vi "Create System Image (Folder).vi"(4 "File and Directory Blacklist":string[](array[string]), 5 "Encryption Passphrase":string, 6 "Overwrite (F)":bool, 7 "Restart Automatically (T)":bool=TRUE, 8 "error in (no error)":errorcluster, 9 "Image Metadata in":T1={"title"="", "description"="", "ID"="", "version"="", "component type"=5} {"component type" items=["standard", "hidden", "system", "unknown", "startup", "image"]}, 10 "Destination Folder":path, 11 "Session in":refnum<k21>) -> (0 "error out":errorcluster, 1 "Image Metadata out":T1={"title"="", "description"="", "ID"="", "version"="", "component type"=5} {"component type" items=["standard", "hidden", "system", "unknown", "startup", "image"]}, 3 "Session out":refnum<k21>)   [LabVIEW 2014, in "nisyscfg.lvlib"]
doc: "Creates a system image folder—a copy of the contents and software on a primary hard drive of a system. You may want to create a system image to restore a system to its original state or to deploy the image to other systems."
uses:
  nisyscfg.lvlib
  Software 1.2.ctl
  Component Type.ctl
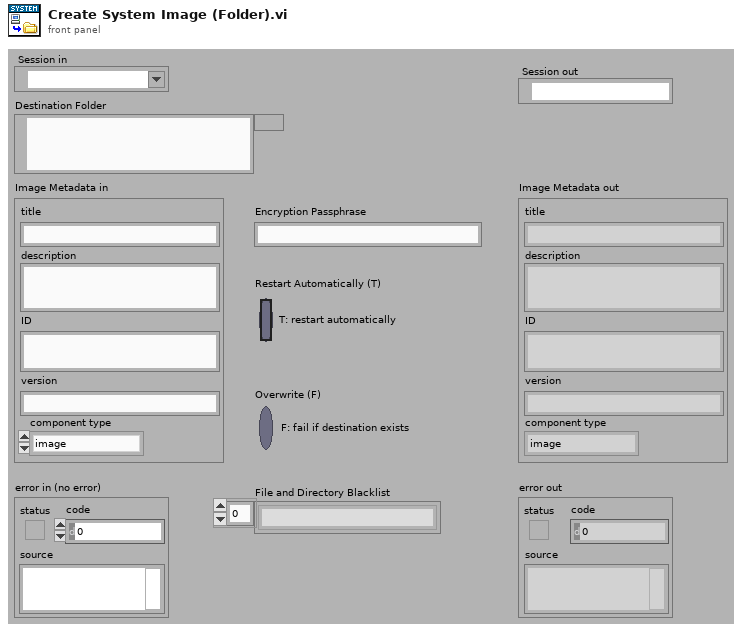
[diagram p1: front panel]
types:
  T1 = typedef "nisyscfg.lvlib/Software 1.2.ctl" = cluster{"title":string, "description":string, "ID":string, "version":string, "component type":T2}
  T2 = typedef "nisyscfg.lvlib/Component Type.ctl" = u32
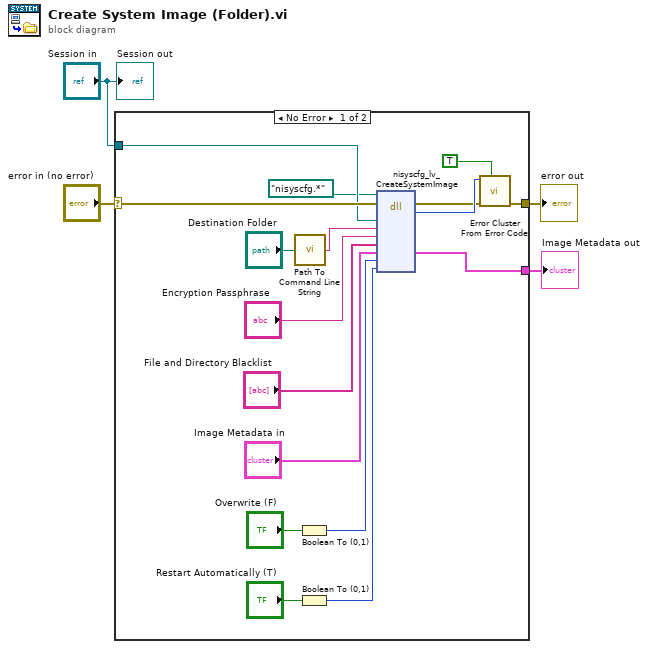
[diagram p0: block diagram]
diagram:
  n1 = case shown="No Error" "error in (no error)" {
    selector: "error in (no error)" -> [w18 w22]
    tunnel: [w21 w22] -> w4
    tunnel: "Session in" -> [w17 _]
    tunnel: [w5 _] -> w1
    frame No Error {
      n2 = call "Path To Command Line String.vi"("path"="Destination Folder") -> ("string"=w7:string)
      n3 = Boolean To (0,1)(Boolean="Overwrite (F)") -> (0, 1=w14:i16)
      n4 = Boolean To (0,1)(Boolean="Restart Automatically (T)") -> (0, 1=w11:i16)
      n5 = dll-call lib="nisyscfg.*" fn="nisyscfg_lv_CreateSystemImage" label="Create System Image"(path in=path "nisyscfg.*", error in=w18, "system"=w17, "localImagePath"=w7, "encryptionPassphrase"="Encryption Passphrase", "blacklist"="File and Directory Blacklist", "imageMetadata"="Image Metadata in", "overwriteIfExists"=w14, "restartAutomatically"=w11) -> (error out=w19:errorcluster, "result"=w20:i32, "imageMetadata"=w5:T1)  [unwired: 7 in, 1 out]
      n6 = call "Error Cluster From Error Code.vi"("show call chain? (False)"=TRUE, "error in (no error)"=w19, "error code (0)"=w20) -> ("error out"=w21:errorcluster)  [unwired: 6 in]
    }
    frame Error {
    }
  }
  "error out" <- w4
  "Image Metadata out" <- w1
  "Session out" <- "Session in"
